vi "GT Set Step Config.vi"(8 "error in (no error)":errorcluster caption="错误输入（无错误）", 9 "pStep":T1, 10 "step":i16, 11 "cardNum":i16) -> (0 "error out":errorcluster caption="错误输出", 1 "pStep out":T1, 3 "function return":i16)   [LabVIEW 2020, in "gts1.lvlib"]
doc: "GT_API GT_SetStepConfig(short cardNum,short step,TStepConfig *pStep);"
uses:
  gts1.lvlib
  dll/32bit/multi_card/gts.dll
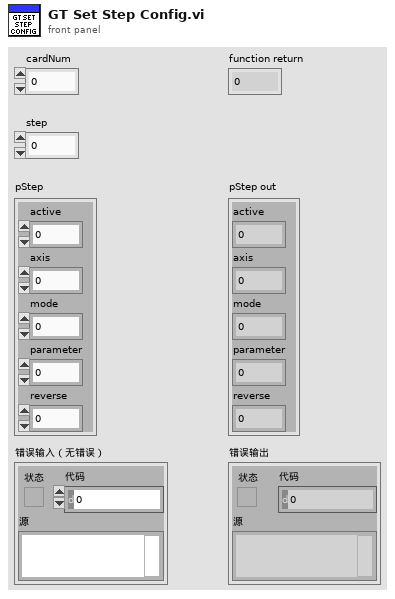
[diagram p1: front panel]
types:
  T1 = cluster{"active":i16, "axis":i16, "mode":i16, "parameter":i16, "reverse":i16}
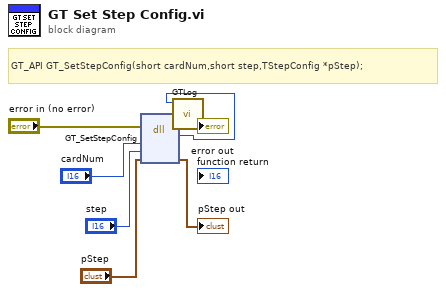
[diagram p0: block diagram]
diagram:
  # "GT_API GT_SetStepConfig(short cardNum,short step,TStepConfig *pStep);"
  n1 = dll-call lib="C:/1228/dll/32bit/multi_card/gts.dll" fn="GT_SetStepConfig"(error in="error in (no error)", "cardNum"="cardNum", "step"="step", "pStep"="pStep") -> (error out=w3:errorcluster, w1:i16, "pStep"=→"pStep out":T1)  [unwired: 4 in, 1 out]
  n2 = call "GTLog.vi"("error in (no error)"=w3, "Numeric"=w1) -> ("error out"=→"error out":errorcluster)  [unwired: 9 in]
